vi "PSS_Telemetry.vi"(10 "Variant":variant) -> (2 "Telemetry_Out":T1={"Register 0"={"PSS_ID"=1, "PSS_Fuse"=2, "PSS_Rev"=3}, "Register 1"={"inhSafe_Out"=TRUE, "nPOR_B1"=FALSE, "nPOR_B0"=TRUE, "nBusPwrGood1"=FALSE, "nBusPwrGood0"=TRUE, "parBoard"=FALSE, "disCMD_B"=TRUE, "disCMD_A"=TRUE, "forceCMD_B"=FALSE, "forceCMD_A"=TRUE, "enOCP"=FALSE, "errRegInPar"=TRUE, "errWatchdog"=FALSE, "enbWatchdog"=TRUE, "staSoftRST"=FALSE, "statusPOR"=TRUE}, "Register 2"={"DetUV_C"=FALSE, "DetUV_B"=FALSE, "DetUV_A"=FALSE, "DetUV"=TRUE, "Conf_A[0]"=FALSE, "Conf_A[1]"=FALSE, "Conf_B[0]"=FALSE, "Conf_B[1]"=FALSE, "SetStatic_A"=FALSE, "SetStatic_B"=FALSE, "SetStatic_C"=FALSE, "SetStatic_D"=FALSE, "SetStatic_E"=FALSE, "SetStatic_F"=FALSE, "SetStatic_G"=FALSE, "SetStatic_H"=FALSE}, "Register 3"={"WDOG_Count"=21, "DISCO_00"=FALSE, "DISCO_01"=FALSE, "DISCO_02"=FALSE, "DISCO_03"=FALSE, "String_ID"=enum."No_String", "ID_Node"=0}, "Register 4"={"Last_VAL_FUNC_A"=enum."Static_Switch", "badFuncCMD_A"=FALSE, "badPulseCMD_A"=FALSE, "errChkSum_A"=TRUE, "errTimeCMD_A"=FALSE, "errParCMD_A"=FALSE, "errStopCMD_A"=FALSE, "enChanCMD_A"=FALSE, "errBusyTeleAddr_A"=FALSE, "errUdefTeleAddr_A"=FALSE, "errParTeleAddr_A"=FALSE, "errStopTeleAddr_A"=FALSE, "enbTeleAddr_A"=FALSE}, "Register_5"={"CMD_A_VALID_CMD_CNT"=0, "CMD_A_BAD_CMD_CNT"=0}, "Register 6"={"Last_VAL_FUNC_B"=enum."Static_Switch", "badFuncCMD_B"=FALSE, "badPulseCMD_B"=FALSE, "errChkSum_B"=FALSE, "errTimeCMD_B"=TRUE, "errParCMD_B"=FALSE, "errStopCMD_B"=FALSE, "enChanCMD_B"=FALSE, "errBusyTeleAddr_B"=FALSE, "errUdefTeleAddr_B"=FALSE, "errParTeleAddr_B"=FALSE, "errStopTeleAddr_B"=FALSE, "enbTeleAddr_B"=FALSE}, "Register_7"={"CMD_B_VALID_CMD_CNT"=0, "CMD_B_BAD_CMD_CNT"=0}, "Register_8"={"CH01_00A_L"=FALSE, "CH01_00A_H"=FALSE, "CH02_00A_L"=FALSE, "CH02_00A_H"=TRUE, "CH03_00A_L"=FALSE, "CH03_00A_H"=FALSE, "CH04_00A_L"=FALSE, "CH04_00A_H"=FALSE, "CH05_00A_L"=FALSE, "CH05_00A_H"=FALSE, "CH06_00A_L"=FALSE, "CH06_00A_H"=FALSE, "CH07_00A_L"=FALSE, "CH07_00A_H"=FALSE, "CH08_00A_L"=FALSE, "CH08_00A_H"=FALSE}, "Register_9"={"CH09_00A_L"=FALSE, "CH09_00A_H"=FALSE, "CH10_00A_L"=FALSE, "CH10_00A_H"=FALSE, "CH11_00A_L"=FALSE, "CH11_00A_H"=FALSE, "CH12_00A_L"=FALSE, "CH12_00A_H"=FALSE, "CH13_00A_L"=FALSE, "CH13_00A_H"=FALSE, "CH14_00A_L"=FALSE, "CH14_00A_H"=FALSE, "CH15_00A_L"=FALSE, "CH15_00A_H"=FALSE, "CH16_00A_L"=TRUE, "CH16_00A_H"=FALSE}, "Register_A"={"CH17_00A_L"=FALSE, "CH17_00A_H"=FALSE, "CH18_00A_L"=FALSE, "CH18_00A_H"=FALSE, "CH19_00A_L"=TRUE, "CH19_00A_H"=FALSE, "CH20_00A_L"=FALSE, "CH20_00A_H"=FALSE, "CH21_00A_L"=FALSE, "CH21_00A_H"=FALSE, "CH22_00A_L"=FALSE, "CH22_00A_H"=FALSE, "CH23_00A_L"=FALSE, "CH23_00A_H"=FALSE, "CH24_00A_L"=FALSE, "CH24_00A_H"=FALSE}, "Register_B"={"CH25_00A_L"=FALSE, "CH25_00A_H"=FALSE, "CH26_00A_L"=FALSE, "CH26_00A_H"=FALSE, "CH27_00A_L"=FALSE, "CH27_00A_H"=FALSE, "CH28_00A_L"=FALSE, "CH28_00A_H"=FALSE, "CH29_00A_L"=FALSE, "CH29_00A_H"=FALSE, "CH30_00A_L"=TRUE, "CH30_00A_H"=FALSE, "CH31_00A_L"=FALSE, "CH31_00A_H"=FALSE, "CH32_00A_L"=FALSE, "CH32_00A_H"=FALSE}, "Register_C"={"CH01_00A_L"=FALSE, "CH01_00A_H"=FALSE, "CH02_00A_L"=FALSE, "CH02_00A_H"=FALSE, "CH03_00A_L"=FALSE, "CH03_00A_H"=FALSE, "CH04_00A_L"=FALSE, "CH04_00A_H"=TRUE, "CH05_00A_L"=FALSE, "CH05_00A_H"=FALSE, "CH06_00A_L"=FALSE, "CH06_00A_H"=FALSE, "CH07_00A_L"=FALSE, "CH07_00A_H"=FALSE, "CH08_00A_L"=FALSE, "CH08_00A_H"=FALSE}, "Register_D"={"CH09_00A_L"=TRUE, "CH09_00A_H"=FALSE, "CH10_00A_L"=FALSE, "CH10_00A_H"=FALSE, "CH11_00A_L"=FALSE, "CH11_00A_H"=FALSE, "CH12_00A_L"=FALSE, "CH12_00A_H"=FALSE, "CH13_00A_L"=FALSE, "CH13_00A_H"=FALSE, "CH14_00A_L"=FALSE, "CH14_00A_H"=FALSE, "CH15_00A_L"=FALSE, "CH15_00A_H"=FALSE, "CH16_00A_L"=FALSE, "CH16_00A_H"=FALSE}, "Register_E"={"CH17_00A_L"=FALSE, "CH17_00A_H"=FALSE, "CH18_00A_L"=FALSE, "CH18_00A_H"=FALSE, "CH19_00A_L"=FALSE, "CH19_00A_H"=FALSE, "CH20_00A_L"=FALSE, "CH20_00A_H"=FALSE, "CH21_00A_L"=TRUE, "CH21_00A_H"=FALSE, "CH22_00A_L"=FALSE, "CH22_00A_H"=FALSE, "CH23_00A_L"=FALSE, "CH23_00A_H"=FALSE, "CH24_00A_L"=FALSE, "CH24_00A_H"=FALSE}, "Register_F"={"CH25_00A_L"=FALSE, "CH25_00A_H"=FALSE, "CH26_00A_L"=FALSE, "CH26_00A_H"=FALSE, "CH27_00A_L"=FALSE, "CH27_00A_H"=FALSE, "CH28_00A_L"=FALSE, "CH28_00A_H"=FALSE, "CH29_00A_L"=FALSE, "CH29_00A_H"=FALSE, "CH30_00A_L"=FALSE, "CH30_00A_H"=FALSE, "CH31_00A_L"=FALSE, "CH31_00A_H"=FALSE, "CH32_00A_L"=FALSE, "CH32_00A_H"=TRUE}, "Raw Digital Telemetry"=[], "Raw Analog MUX_1"=[], "Raw Analog MUX_2"=[], "Raw Analog MUX_3"=[], "Raw Analog MUX_4"=[], "Raw Analog MUX_5"=[], "Timeout"=TRUE, "Scaled_Analog"=[], "Full_Switch_State"=[{"HS_Switch"=FALSE, "LS_Switch"=FALSE, "HS_OCP"=FALSE, "LS_OCP"=FALSE, "HS_Current"=0.0, "LS_Current"=0.0, "Current_Rating"=0.0, "Switch_Cfg"=enum."Static", "R_Load"=0.0}, {"HS_Switch"=FALSE, "LS_Switch"=FALSE, "HS_OCP"=FALSE, "LS_OCP"=FALSE, "HS_Current"=0.0, "LS_Current"=0.0, "Current_Rating"=0.0, "Switch_Cfg"=enum."Static", "R_Load"=0.0}, {"HS_Switch"=FALSE, "LS_Switch"=FALSE, "HS_OCP"=FALSE, "LS_OCP"=FALSE, "HS_Current"=0.0, "LS_Current"=0.0, "Current_Rating"=0.0, "Switch_Cfg"=enum."Static", "R_Load"=0.0}, {"HS_Switch"=FALSE, "LS_Switch"=FALSE, "HS_OCP"=FALSE, "LS_OCP"=FALSE, "HS_Current"=0.0, "LS_Current"=0.0, "Current_Rating"=0.0, "Switch_Cfg"=enum."Static", "R_Load"=0.0}, {"HS_Switch"=FALSE, "LS_Switch"=FALSE, "HS_OCP"=FALSE, "LS_OCP"=FALSE, "HS_Current"=0.0, "LS_Current"=0.0, "Current_Rating"=0.0, "Switch_Cfg"=enum."Static", "R_Load"=0.0}, {"HS_Switch"=FALSE, "LS_Switch"=FALSE, "HS_OCP"=FALSE, "LS_OCP"=FALSE, "HS_Current"=0.0, "LS_Current"=0.0, "Current_Rating"=0.0, "Switch_Cfg"=enum."Static", "R_Load"=0.0}, {"HS_Switch"=FALSE, "LS_Switch"=FALSE, "HS_OCP"=FALSE, "LS_OCP"=FALSE, "HS_Current"=0.0, "LS_Current"=0.0, "Current_Rating"=0.0, "Switch_Cfg"=enum."Static", "R_Load"=0.0}, {"HS_Switch"=FALSE, "LS_Switch"=FALSE, "HS_OCP"=FALSE, "LS_OCP"=FALSE, "HS_Current"=0.0, "LS_Current"=0.0, "Current_Rating"=0.0, "Switch_Cfg"=enum."Static", "R_Load"=0.0}, {"HS_Switch"=FALSE, "LS_Switch"=FALSE, "HS_OCP"=FALSE, "LS_OCP"=FALSE, "HS_Current"=0.0, "LS_Current"=0.0, "Current_Rating"=0.0, "Switch_Cfg"=enum."Static", "R_Load"=0.0}, {"HS_Switch"=FALSE, "LS_Switch"=FALSE, "HS_OCP"=FALSE, "LS_OCP"=FALSE, "HS_Current"=0.0, "LS_Current"=0.0, "Current_Rating"=0.0, "Switch_Cfg"=enum."Static", "R_Load"=0.0}, {"HS_Switch"=FALSE, "LS_Switch"=FALSE, "HS_OCP"=FALSE, "LS_OCP"=FALSE, "HS_Current"=0.0, "LS_Current"=0.0, "Current_Rating"=0.0, "Switch_Cfg"=enum."Static", "R_Load"=0.0}, {"HS_Switch"=FALSE, "LS_Switch"=FALSE, "HS_OCP"=FALSE, "LS_OCP"=FALSE, "HS_Current"=0.0, "LS_Current"=0.0, "Current_Rating"=0.0, "Switch_Cfg"=enum."Static", "R_Load"=0.0}, {"HS_Switch"=FALSE, "LS_Switch"=FALSE, "HS_OCP"=FALSE, "LS_OCP"=FALSE, "HS_Current"=0.0, "LS_Current"=0.0, "Current_Rating"=0.0, "Switch_Cfg"=enum."Static", "R_Load"=0.0}, {"HS_Switch"=FALSE, "LS_Switch"=FALSE, "HS_OCP"=FALSE, "LS_OCP"=FALSE, "HS_Current"=0.0, "LS_Current"=0.0, "Current_Rating"=0.0, "Switch_Cfg"=enum."Static", "R_Load"=0.0}, {"HS_Switch"=FALSE, "LS_Switch"=FALSE, "HS_OCP"=FALSE, "LS_OCP"=FALSE, "HS_Current"=0.0, "LS_Current"=0.0, "Current_Rating"=0.0, "Switch_Cfg"=enum."Static", "R_Load"=0.0}, {"HS_Switch"=FALSE, "LS_Switch"=FALSE, "HS_OCP"=FALSE, "LS_OCP"=FALSE, "HS_Current"=0.0, "LS_Current"=0.0, "Current_Rating"=0.0, "Switch_Cfg"=enum."Static", "R_Load"=0.0}, {"HS_Switch"=FALSE, "LS_Switch"=FALSE, "HS_OCP"=FALSE, "LS_OCP"=FALSE, "HS_Current"=0.0, "LS_Current"=0.0, "Current_Rating"=0.0, "Switch_Cfg"=enum."Static", "R_Load"=0.0}, {"HS_Switch"=FALSE, "LS_Switch"=FALSE, "HS_OCP"=FALSE, "LS_OCP"=FALSE, "HS_Current"=0.0, "LS_Current"=0.0, "Current_Rating"=0.0, "Switch_Cfg"=enum."Static", "R_Load"=0.0}, {"HS_Switch"=FALSE, "LS_Switch"=FALSE, "HS_OCP"=FALSE, "LS_OCP"=FALSE, "HS_Current"=0.0, "LS_Current"=0.0, "Current_Rating"=0.0, "Switch_Cfg"=enum."Static", "R_Load"=0.0}, {"HS_Switch"=FALSE, "LS_Switch"=FALSE, "HS_OCP"=FALSE, "LS_OCP"=FALSE, "HS_Current"=0.0, "LS_Current"=0.0, "Current_Rating"=0.0, "Switch_Cfg"=enum."Static", "R_Load"=0.0}, {"HS_Switch"=FALSE, "LS_Switch"=FALSE, "HS_OCP"=FALSE, "LS_OCP"=FALSE, "HS_Current"=0.0, "LS_Current"=0.0, "Current_Rating"=0.0, "Switch_Cfg"=enum."Static", "R_Load"=0.0}, {"HS_Switch"=FALSE, "LS_Switch"=FALSE, "HS_OCP"=FALSE, "LS_OCP"=FALSE, "HS_Current"=0.0, "LS_Current"=0.0, "Current_Rating"=0.0, "Switch_Cfg"=enum."Static", "R_Load"=0.0}, {"HS_Switch"=FALSE, "LS_Switch"=FALSE, "HS_OCP"=FALSE, "LS_OCP"=FALSE, "HS_Current"=0.0, "LS_Current"=0.0, "Current_Rating"=0.0, "Switch_Cfg"=enum."Static", "R_Load"=0.0}, {"HS_Switch"=FALSE, "LS_Switch"=FALSE, "HS_OCP"=FALSE, "LS_OCP"=FALSE, "HS_Current"=0.0, "LS_Current"=0.0, "Current_Rating"=0.0, "Switch_Cfg"=enum."Static", "R_Load"=0.0}, {"HS_Switch"=FALSE, "LS_Switch"=FALSE, "HS_OCP"=FALSE, "LS_OCP"=FALSE, "HS_Current"=0.0, "LS_Current"=0.0, "Current_Rating"=0.0, "Switch_Cfg"=enum."Static", "R_Load"=0.0}, {"HS_Switch"=FALSE, "LS_Switch"=FALSE, "HS_OCP"=FALSE, "LS_OCP"=FALSE, "HS_Current"=0.0, "LS_Current"=0.0, "Current_Rating"=0.0, "Switch_Cfg"=enum."Static", "R_Load"=0.0}, {"HS_Switch"=FALSE, "LS_Switch"=FALSE, "HS_OCP"=FALSE, "LS_OCP"=FALSE, "HS_Current"=0.0, "LS_Current"=0.0, "Current_Rating"=0.0, "Switch_Cfg"=enum."Static", "R_Load"=0.0}, {"HS_Switch"=FALSE, "LS_Switch"=FALSE, "HS_OCP"=FALSE, "LS_OCP"=FALSE, "HS_Current"=0.0, "LS_Current"=0.0, "Current_Rating"=0.0, "Switch_Cfg"=enum."Static", "R_Load"=0.0}, {"HS_Switch"=FALSE, "LS_Switch"=FALSE, "HS_OCP"=FALSE, "LS_OCP"=FALSE, "HS_Current"=0.0, "LS_Current"=0.0, "Current_Rating"=0.0, "Switch_Cfg"=enum."Static", "R_Load"=0.0}, {"HS_Switch"=FALSE, "LS_Switch"=FALSE, "HS_OCP"=FALSE, "LS_OCP"=FALSE, "HS_Current"=0.0, "LS_Current"=0.0, "Current_Rating"=0.0, "Switch_Cfg"=enum."Static", "R_Load"=0.0}, {"HS_Switch"=FALSE, "LS_Switch"=FALSE, "HS_OCP"=FALSE, "LS_OCP"=FALSE, "HS_Current"=0.0, "LS_Current"=0.0, "Current_Rating"=0.0, "Switch_Cfg"=enum."Static", "R_Load"=0.0}, {"HS_Switch"=FALSE, "LS_Switch"=FALSE, "HS_OCP"=FALSE, "LS_OCP"=FALSE, "HS_Current"=0.0, "LS_Current"=0.0, "Current_Rating"=0.0, "Switch_Cfg"=enum."Static", "R_Load"=0.0}]} {"Register 3"."ID_Node" format="%02x"; "Register 3"."WDOG_Count" format="%02x"; "Register 0"."PSS_Rev" format="%02x"; "Register 0"."PSS_Fuse" format="%02x"; "Register 0"."PSS_ID" format="%02x"})   [LabVIEW 2019, in "Variant Parser.lvlib" / "Variant Parser.lvclass"]
uses:
  Library/Variant Parser.lvclass
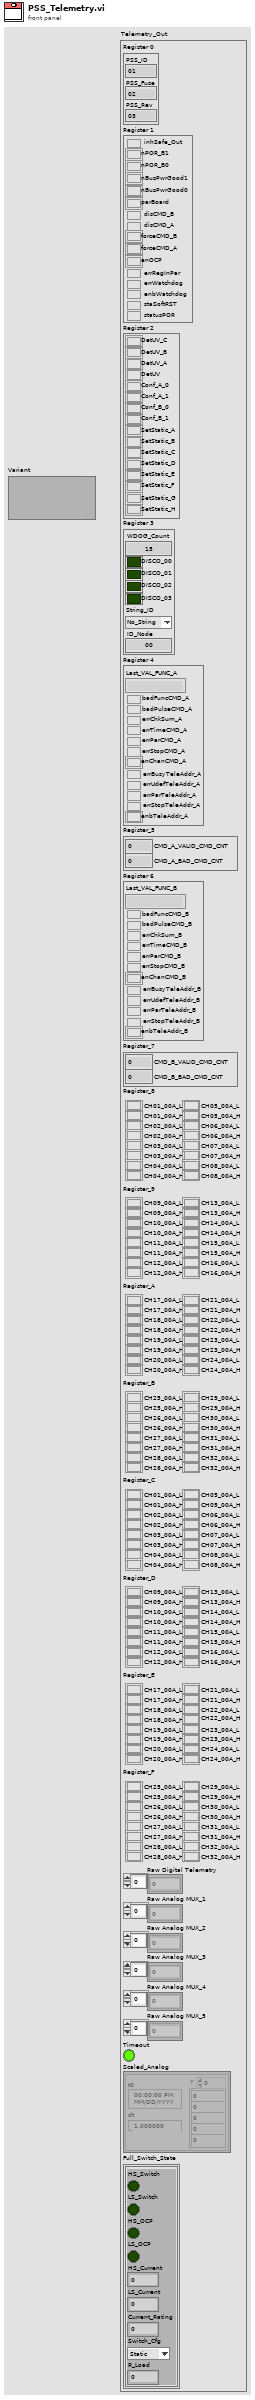
[diagram p1: front panel]
types:
  T1 = cluster{"Register 0":cluster{"PSS_ID":u8, "PSS_Fuse":u8, "PSS_Rev":u8}, "Register 1":cluster{"inhSafe_Out":bool, "nPOR_B1":bool, "nPOR_B0":bool, "nBusPwrGood1":bool, "nBusPwrGood0":bool, "parBoard":bool, "disCMD_B":bool, "disCMD_A":bool, "forceCMD_B":bool, "forceCMD_A":bool, "enOCP":bool, "errRegInPar":bool, "errWatchdog":bool, "enbWatchdog":bool, "staSoftRST":bool, "statusPOR":bool}, "Register 2":cluster{"DetUV_C":bool, "DetUV_B":bool, "DetUV_A":bool, "DetUV":bool, "Conf_A[0]":bool, "Conf_A[1]":bool, "Conf_B[0]":bool, "Conf_B[1]":bool, "SetStatic_A":bool, "SetStatic_B":bool, "SetStatic_C":bool, "SetStatic_D":bool, "SetStatic_E":bool, "SetStatic_F":bool, "SetStatic_G":bool, "SetStatic_H":bool}, "Register 3":cluster{"WDOG_Count":u8, "DISCO_00":bool, "DISCO_01":bool, "DISCO_02":bool, "DISCO_03":bool, "String_ID":enum16{"No_String", "String_A", "String_B", "Both_Strings"}, "ID_Node":u8}, "Register 4":cluster{"Last_VAL_FUNC_A":enum16{"Static_Switch", "Dynamic_Switch", "IO_Command", "Housekeeping", "Miscellaneous", "No_Operation", "Bad_Function"}, "badFuncCMD_A":bool, "badPulseCMD_A":bool, "errChkSum_A":bool, "errTimeCMD_A":bool, "errParCMD_A":bool, "errStopCMD_A":bool, "enChanCMD_A":bool, "errBusyTeleAddr_A":bool, "errUdefTeleAddr_A":bool, "errParTeleAddr_A":bool, "errStopTeleAddr_A":bool, "enbTeleAddr_A":bool}, "Register_5":cluster{"CMD_A_VALID_CMD_CNT":u8, "CMD_A_BAD_CMD_CNT":u8}, "Register 6":cluster{"Last_VAL_FUNC_B":enum16{"Static_Switch", "Dynamic_Switch", "IO_Command", "Housekeeping", "Miscellaneous", "No_Operation", "Bad_Function"}, "badFuncCMD_B":bool, "badPulseCMD_B":bool, "errChkSum_B":bool, "errTimeCMD_B":bool, "errParCMD_B":bool, "errStopCMD_B":bool, "enChanCMD_B":bool, "errBusyTeleAddr_B":bool, "errUdefTeleAddr_B":bool, "errParTeleAddr_B":bool, "errStopTeleAddr_B":bool, "enbTeleAddr_B":bool}, "Register_7":cluster{"CMD_B_VALID_CMD_CNT":u8, "CMD_B_BAD_CMD_CNT":u8}, "Register_8":cluster{"CH01_00A_L":bool, "CH01_00A_H":bool, "CH02_00A_L":bool, "CH02_00A_H":bool, "CH03_00A_L":bool, "CH03_00A_H":bool, "CH04_00A_L":bool, "CH04_00A_H":bool, "CH05_00A_L":bool, "CH05_00A_H":bool, "CH06_00A_L":bool, "CH06_00A_H":bool, "CH07_00A_L":bool, "CH07_00A_H":bool, "CH08_00A_L":bool, "CH08_00A_H":bool}, "Register_9":cluster{"CH09_00A_L":bool, "CH09_00A_H":bool, "CH10_00A_L":bool, "CH10_00A_H":bool, "CH11_00A_L":bool, "CH11_00A_H":bool, "CH12_00A_L":bool, "CH12_00A_H":bool, "CH13_00A_L":bool, "CH13_00A_H":bool, "CH14_00A_L":bool, "CH14_00A_H":bool, "CH15_00A_L":bool, "CH15_00A_H":bool, "CH16_00A_L":bool, "CH16_00A_H":bool}, "Register_A":cluster{"CH17_00A_L":bool, "CH17_00A_H":bool, "CH18_00A_L":bool, "CH18_00A_H":bool, "CH19_00A_L":bool, "CH19_00A_H":bool, "CH20_00A_L":bool, "CH20_00A_H":bool, "CH21_00A_L":bool, "CH21_00A_H":bool, "CH22_00A_L":bool, "CH22_00A_H":bool, "CH23_00A_L":bool, "CH23_00A_H":bool, "CH24_00A_L":bool, "CH24_00A_H":bool}, "Register_B":cluster{"CH25_00A_L":bool, "CH25_00A_H":bool, "CH26_00A_L":bool, "CH26_00A_H":bool, "CH27_00A_L":bool, "CH27_00A_H":bool, "CH28_00A_L":bool, "CH28_00A_H":bool, "CH29_00A_L":bool, "CH29_00A_H":bool, "CH30_00A_L":bool, "CH30_00A_H":bool, "CH31_00A_L":bool, "CH31_00A_H":bool, "CH32_00A_L":bool, "CH32_00A_H":bool}, "Register_C":cluster{"CH01_00A_L":bool, "CH01_00A_H":bool, "CH02_00A_L":bool, "CH02_00A_H":bool, "CH03_00A_L":bool, "CH03_00A_H":bool, "CH04_00A_L":bool, "CH04_00A_H":bool, "CH05_00A_L":bool, "CH05_00A_H":bool, "CH06_00A_L":bool, "CH06_00A_H":bool, "CH07_00A_L":bool, "CH07_00A_H":bool, "CH08_00A_L":bool, "CH08_00A_H":bool}, "Register_D":cluster{"CH09_00A_L":bool, "CH09_00A_H":bool, "CH10_00A_L":bool, "CH10_00A_H":bool, "CH11_00A_L":bool, "CH11_00A_H":bool, "CH12_00A_L":bool, "CH12_00A_H":bool, "CH13_00A_L":bool, "CH13_00A_H":bool, "CH14_00A_L":bool, "CH14_00A_H":bool, "CH15_00A_L":bool, "CH15_00A_H":bool, "CH16_00A_L":bool, "CH16_00A_H":bool}, "Register_E":cluster{"CH17_00A_L":bool, "CH17_00A_H":bool, "CH18_00A_L":bool, "CH18_00A_H":bool, "CH19_00A_L":bool, "CH19_00A_H":bool, "CH20_00A_L":bool, "CH20_00A_H":bool, "CH21_00A_L":bool, "CH21_00A_H":bool, "CH22_00A_L":bool, "CH22_00A_H":bool, "CH23_00A_L":bool, "CH23_00A_H":bool, "CH24_00A_L":bool, "CH24_00A_H":bool}, "Register_F":cluster{"CH25_00A_L":bool, "CH25_00A_H":bool, "CH26_00A_L":bool, "CH26_00A_H":bool, "CH27_00A_L":bool, "CH27_00A_H":bool, "CH28_00A_L":bool, "CH28_00A_H":bool, "CH29_00A_L":bool, "CH29_00A_H":bool, "CH30_00A_L":bool, "CH30_00A_H":bool, "CH31_00A_L":bool, "CH31_00A_H":bool, "CH32_00A_L":bool, "CH32_00A_H":bool}, "Raw Digital Telemetry":u16[], "Raw Analog MUX_1":u16[], "Raw Analog MUX_2":u16[], "Raw Analog MUX_3":u16[], "Raw Analog MUX_4":u16[], "Raw Analog MUX_5":u16[], "Timeout":bool, "Scaled_Analog":waveform(dbl)[], "Full_Switch_State":cluster{"HS_Switch":bool, "LS_Switch":bool, "HS_OCP":bool, "LS_OCP":bool, "HS_Current":dbl, "LS_Current":dbl, "Current_Rating":dbl, "Switch_Cfg":enum16{"Static", "Pulsed", "Safety", "Critical"}, "R_Load":dbl}[]}
  T2 = cluster{"Register 0":cluster{"PSS_ID":u8, "PSS_Fuse":u8, "PSS_Rev":u8}, "Register 1":cluster{"inhSafe_Out":bool, "nPOR_B1":bool, "nPOR_B0":bool, "nBusPwrGood1":bool, "nBusPwrGood0":bool, "parBoard":bool, "disCMD_B":bool, "disCMD_A":bool, "forceCMD_B":bool, "forceCMD_A":bool, "enOCP":bool, "errRegInPar":bool, "errWatchdog":bool, "enbWatchdog":bool, "staSoftRST":bool, "statusPOR":bool}, "Register 2":cluster{"DetUV_C":bool, "DetUV_B":bool, "DetUV_A":bool, "DetUV":bool, "Conf_A[0]":bool, "Conf_A[1]":bool, "Conf_B[0]":bool, "Conf_B[1]":bool, "SetStatic_A":bool, "SetStatic_B":bool, "SetStatic_C":bool, "SetStatic_D":bool, "SetStatic_E":bool, "SetStatic_F":bool, "SetStatic_G":bool, "SetStatic_H":bool}, "Register 3":cluster{"WDOG_Count":u8, "DISCO_00":bool, "DISCO_01":bool, "DISCO_02":bool, "DISCO_03":bool, "String_ID":enum16{"No_String", "String_A", "String_B", "Both_Strings"}, "ID_Node":u8}, "Register 4":cluster{"Last_VAL_FUNC_A":enum16{"Static_Switch", "Dynamic_Switch", "IO_Command", "Housekeeping", "Miscellaneous", "No_Operation", "Bad_Function"}, "badFuncCMD_A":bool, "badPulseCMD_A":bool, "errChkSum_A":bool, "errTimeCMD_A":bool, "errParCMD_A":bool, "errStopCMD_A":bool, "enChanCMD_A":bool, "errBusyTeleAddr_A":bool, "errUdefTeleAddr_A":bool, "errParTeleAddr_A":bool, "errStopTeleAddr_A":bool, "enbTeleAddr_A":bool}, "Register_5":cluster{"CMD_A_VALID_CMD_CNT":u8, "CMD_A_BAD_CMD_CNT":u8}, "Register 6":cluster{"Last_VAL_FUNC_B":enum16{"Static_Switch", "Dynamic_Switch", "IO_Command", "Housekeeping", "Miscellaneous", "No_Operation", "Bad_Function"}, "badFuncCMD_B":bool, "badPulseCMD_B":bool, "errChkSum_B":bool, "errTimeCMD_B":bool, "errParCMD_B":bool, "errStopCMD_B":bool, "enChanCMD_B":bool, "errBusyTeleAddr_B":bool, "errUdefTeleAddr_B":bool, "errParTeleAddr_B":bool, "errStopTeleAddr_B":bool, "enbTeleAddr_B":bool}, "Register_7":cluster{"CMD_B_VALID_CMD_CNT":u8, "CMD_B_BAD_CMD_CNT":u8}, "Register_8":cluster{"CH01_00A_L":bool, "CH01_00A_H":bool, "CH02_00A_L":bool, "CH02_00A_H":bool, "CH03_00A_L":bool, "CH03_00A_H":bool, "CH04_00A_L":bool, "CH04_00A_H":bool, "CH05_00A_L":bool, "CH05_00A_H":bool, "CH06_00A_L":bool, "CH06_00A_H":bool, "CH07_00A_L":bool, "CH07_00A_H":bool, "CH08_00A_L":bool, "CH08_00A_H":bool}, "Register_9":cluster{"CH09_00A_L":bool, "CH09_00A_H":bool, "CH10_00A_L":bool, "CH10_00A_H":bool, "CH11_00A_L":bool, "CH11_00A_H":bool, "CH12_00A_L":bool, "CH12_00A_H":bool, "CH13_00A_L":bool, "CH13_00A_H":bool, "CH14_00A_L":bool, "CH14_00A_H":bool, "CH15_00A_L":bool, "CH15_00A_H":bool, "CH16_00A_L":bool, "CH16_00A_H":bool}, "Register_A":cluster{"CH17_00A_L":bool, "CH17_00A_H":bool, "CH18_00A_L":bool, "CH18_00A_H":bool, "CH19_00A_L":bool, "CH19_00A_H":bool, "CH20_00A_L":bool, "CH20_00A_H":bool, "CH21_00A_L":bool, "CH21_00A_H":bool, "CH22_00A_L":bool, "CH22_00A_H":bool, "CH23_00A_L":bool, "CH23_00A_H":bool, "CH24_00A_L":bool, "CH24_00A_H":bool}, "Register_B":cluster{"CH25_00A_L":bool, "CH25_00A_H":bool, "CH26_00A_L":bool, "CH26_00A_H":bool, "CH27_00A_L":bool, "CH27_00A_H":bool, "CH28_00A_L":bool, "CH28_00A_H":bool, "CH29_00A_L":bool, "CH29_00A_H":bool, "CH30_00A_L":bool, "CH30_00A_H":bool, "CH31_00A_L":bool, "CH31_00A_H":bool, "CH32_00A_L":bool, "CH32_00A_H":bool}, "Register_C":cluster{"CH01_00A_L":bool, "CH01_00A_H":bool, "CH02_00A_L":bool, "CH02_00A_H":bool, "CH03_00A_L":bool, "CH03_00A_H":bool, "CH04_00A_L":bool, "CH04_00A_H":bool, "CH05_00A_L":bool, "CH05_00A_H":bool, "CH06_00A_L":bool, "CH06_00A_H":bool, "CH07_00A_L":bool, "CH07_00A_H":bool, "CH08_00A_L":bool, "CH08_00A_H":bool}, "Register_D":cluster{"CH09_00A_L":bool, "CH09_00A_H":bool, "CH10_00A_L":bool, "CH10_00A_H":bool, "CH11_00A_L":bool, "CH11_00A_H":bool, "CH12_00A_L":bool, "CH12_00A_H":bool, "CH13_00A_L":bool, "CH13_00A_H":bool, "CH14_00A_L":bool, "CH14_00A_H":bool, "CH15_00A_L":bool, "CH15_00A_H":bool, "CH16_00A_L":bool, "CH16_00A_H":bool}, "Register_E":cluster{"CH17_00A_L":bool, "CH17_00A_H":bool, "CH18_00A_L":bool, "CH18_00A_H":bool, "CH19_00A_L":bool, "CH19_00A_H":bool, "CH20_00A_L":bool, "CH20_00A_H":bool, "CH21_00A_L":bool, "CH21_00A_H":bool, "CH22_00A_L":bool, "CH22_00A_H":bool, "CH23_00A_L":bool, "CH23_00A_H":bool, "CH24_00A_L":bool, "CH24_00A_H":bool}, "Register_F":cluster{"CH25_00A_L":bool, "CH25_00A_H":bool, "CH26_00A_L":bool, "CH26_00A_H":bool, "CH27_00A_L":bool, "CH27_00A_H":bool, "CH28_00A_L":bool, "CH28_00A_H":bool, "CH29_00A_L":bool, "CH29_00A_H":bool, "CH30_00A_L":bool, "CH30_00A_H":bool, "CH31_00A_L":bool, "CH31_00A_H":bool, "CH32_00A_L":bool, "CH32_00A_H":bool}, "Raw Digital Telemetry":u16[], "Raw Analog MUX_1":u16[], "Raw Analog MUX_2":u16[], "Raw Analog MUX_3":u16[], "Raw Analog MUX_4":u16[], "Raw Analog MUX_5":u16[], "Timeout":bool, "Scaled_Analog":waveform(dbl)[], "Full_Switch_State":cluster{"HS_Switch":bool, "LS_Switch":bool, "HS_OCP":bool, "LS_OCP":bool, "HS_Current":dbl, "LS_Current":dbl, "Current_Rating":dbl, "Switch_Cfg":enum16{"Static", "Pulsed", "Safety", "Critical"}}[]}
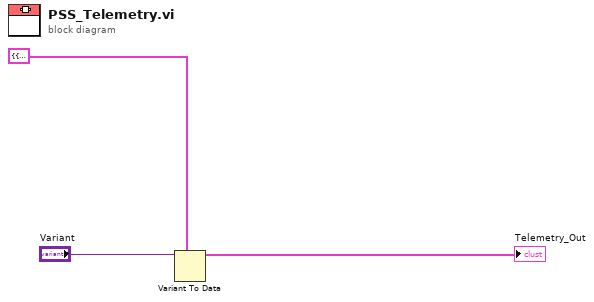
[diagram p0: block diagram]
diagram:
  n1 = Variant To Data(type=T2 {"Register 0"={"PSS_ID"=0, "PSS_Fuse"=0, "PSS_Rev"=0}, "Register 1"={"inhSafe_Out"=FALSE, "nPOR_B1"=FALSE, "nPOR_B0"=FALSE, "nBusPwrGood1"=FALSE, "nBusPwrGood0"=FALSE, "parBoard"=FALSE, "disCMD_B"=FALSE, "disCMD_A"=FALSE, "forceCMD_B"=FALSE, "forceCMD_A"=FALSE, "enOCP"=FALSE, "errRegInPar"=FALSE, "errWatchdog"=FALSE, "enbWatchdog"=FALSE, "staSoftRST"=FALSE, "statusPOR"=FALSE}, "Register 2"={"DetUV_C"=FALSE, "DetUV_B"=FALSE, "DetUV_A"=FALSE, "DetUV"=FALSE, "Conf_A[0]"=FALSE, "Conf_A[1]"=FALSE, "Conf_B[0]"=FALSE, "Conf_B[1]"=FALSE, "SetStatic_A"=FALSE, "SetStatic_B"=FALSE, "SetStatic_C"=FALSE, "SetStatic_D"=FALSE, "SetStatic_E"=FALSE, "SetStatic_F"=FALSE, "SetStatic_G"=FALSE, "SetStatic_H"=FALSE}, "Register 3"={"WDOG_Count"=0, "DISCO_00"=FALSE, "DISCO_01"=FALSE, "DISCO_02"=FALSE, "DISCO_03"=FALSE, "String_ID"=enum."No_String", "ID_Node"=0}, "Register 4"={"Last_VAL_FUNC_A"=enum."Static_Switch", "badFuncCMD_A"=FALSE, "badPulseCMD_A"=FALSE, "errChkSum_A"=FALSE, "errTimeCMD_A"=FALSE, "errParCMD_A"=FALSE, "errStopCMD_A"=FALSE, "enChanCMD_A"=FALSE, "errBusyTeleAddr_A"=FALSE, "errUdefTeleAddr_A"=FALSE, "errParTeleAddr_A"=FALSE, "errStopTeleAddr_A"=FALSE, "enbTeleAddr_A"=FALSE}, "Register_5"={"CMD_A_VALID_CMD_CNT"=0, "CMD_A_BAD_CMD_CNT"=0}, "Register 6"={"Last_VAL_FUNC_B"=enum."Static_Switch", "badFuncCMD_B"=FALSE, "badPulseCMD_B"=FALSE, "errChkSum_B"=FALSE, "errTimeCMD_B"=FALSE, "errParCMD_B"=FALSE, "errStopCMD_B"=FALSE, "enChanCMD_B"=FALSE, "errBusyTeleAddr_B"=FALSE, "errUdefTeleAddr_B"=FALSE, "errParTeleAddr_B"=FALSE, "errStopTeleAddr_B"=FALSE, "enbTeleAddr_B"=FALSE}, "Register_7"={"CMD_B_VALID_CMD_CNT"=0, "CMD_B_BAD_CMD_CNT"=0}, "Register_8"={"CH01_00A_L"=FALSE, "CH01_00A_H"=FALSE, "CH02_00A_L"=FALSE, "CH02_00A_H"=FALSE, "CH03_00A_L"=FALSE, "CH03_00A_H"=FALSE, "CH04_00A_L"=FALSE, "CH04_00A_H"=FALSE, "CH05_00A_L"=FALSE, "CH05_00A_H"=FALSE, "CH06_00A_L"=FALSE, "CH06_00A_H"=FALSE, "CH07_00A_L"=FALSE, "CH07_00A_H"=FALSE, "CH08_00A_L"=FALSE, "CH08_00A_H"=FALSE}, "Register_9"={"CH09_00A_L"=FALSE, "CH09_00A_H"=FALSE, "CH10_00A_L"=FALSE, "CH10_00A_H"=FALSE, "CH11_00A_L"=FALSE, "CH11_00A_H"=FALSE, "CH12_00A_L"=FALSE, "CH12_00A_H"=FALSE, "CH13_00A_L"=FALSE, "CH13_00A_H"=FALSE, "CH14_00A_L"=FALSE, "CH14_00A_H"=FALSE, "CH15_00A_L"=FALSE, "CH15_00A_H"=FALSE, "CH16_00A_L"=FALSE, "CH16_00A_H"=FALSE}, "Register_A"={"CH17_00A_L"=FALSE, "CH17_00A_H"=FALSE, "CH18_00A_L"=FALSE, "CH18_00A_H"=FALSE, "CH19_00A_L"=FALSE, "CH19_00A_H"=FALSE, "CH20_00A_L"=FALSE, "CH20_00A_H"=FALSE, "CH21_00A_L"=FALSE, "CH21_00A_H"=FALSE, "CH22_00A_L"=FALSE, "CH22_00A_H"=FALSE, "CH23_00A_L"=FALSE, "CH23_00A_H"=FALSE, "CH24_00A_L"=FALSE, "CH24_00A_H"=FALSE}, "Register_B"={"CH25_00A_L"=FALSE, "CH25_00A_H"=FALSE, "CH26_00A_L"=FALSE, "CH26_00A_H"=FALSE, "CH27_00A_L"=FALSE, "CH27_00A_H"=FALSE, "CH28_00A_L"=FALSE, "CH28_00A_H"=FALSE, "CH29_00A_L"=FALSE, "CH29_00A_H"=FALSE, "CH30_00A_L"=FALSE, "CH30_00A_H"=FALSE, "CH31_00A_L"=FALSE, "CH31_00A_H"=FALSE, "CH32_00A_L"=FALSE, "CH32_00A_H"=FALSE}, "Register_C"={"CH01_00A_L"=FALSE, "CH01_00A_H"=FALSE, "CH02_00A_L"=FALSE, "CH02_00A_H"=FALSE, "CH03_00A_L"=FALSE, "CH03_00A_H"=FALSE, "CH04_00A_L"=FALSE, "CH04_00A_H"=FALSE, "CH05_00A_L"=FALSE, "CH05_00A_H"=FALSE, "CH06_00A_L"=FALSE, "CH06_00A_H"=FALSE, "CH07_00A_L"=FALSE, "CH07_00A_H"=FALSE, "CH08_00A_L"=FALSE, "CH08_00A_H"=FALSE}, "Register_D"={"CH09_00A_L"=FALSE, "CH09_00A_H"=FALSE, "CH10_00A_L"=FALSE, "CH10_00A_H"=FALSE, "CH11_00A_L"=FALSE, "CH11_00A_H"=FALSE, "CH12_00A_L"=FALSE, "CH12_00A_H"=FALSE, "CH13_00A_L"=FALSE, "CH13_00A_H"=FALSE, "CH14_00A_L"=FALSE, "CH14_00A_H"=FALSE, "CH15_00A_L"=FALSE, "CH15_00A_H"=FALSE, "CH16_00A_L"=FALSE, "CH16_00A_H"=FALSE}, "Register_E"={"CH17_00A_L"=FALSE, "CH17_00A_H"=FALSE, "CH18_00A_L"=FALSE, "CH18_00A_H"=FALSE, "CH19_00A_L"=FALSE, "CH19_00A_H"=FALSE, "CH20_00A_L"=FALSE, "CH20_00A_H"=FALSE, "CH21_00A_L"=FALSE, "CH21_00A_H"=FALSE, "CH22_00A_L"=FALSE, "CH22_00A_H"=FALSE, "CH23_00A_L"=FALSE, "CH23_00A_H"=FALSE, "CH24_00A_L"=FALSE, "CH24_00A_H"=FALSE}, "Register_F"={"CH25_00A_L"=FALSE, "CH25_00A_H"=FALSE, "CH26_00A_L"=FALSE, "CH26_00A_H"=FALSE, "CH27_00A_L"=FALSE, "CH27_00A_H"=FALSE, "CH28_00A_L"=FALSE, "CH28_00A_H"=FALSE, "CH29_00A_L"=FALSE, "CH29_00A_H"=FALSE, "CH30_00A_L"=FALSE, "CH30_00A_H"=FALSE, "CH31_00A_L"=FALSE, "CH31_00A_H"=FALSE, "CH32_00A_L"=FALSE, "CH32_00A_H"=FALSE}, "Raw Digital Telemetry"=[], "Raw Analog MUX_1"=[], "Raw Analog MUX_2"=[], "Raw Analog MUX_3"=[], "Raw Analog MUX_4"=[], "Raw Analog MUX_5"=[], "Timeout"=FALSE, "Scaled_Analog"=[], "Full_Switch_State"=[]} ("data"), Variant="Variant") -> (data=→"Telemetry_Out":T2)  [unwired: 1 in, 1 out]
